vi "Read_Electrical_Variables.vi"(8 "error in (no error)":errorcluster, 11 "Modbus master in":refnum<class "Modbus Master.lvclass">) -> (0 "error out":errorcluster, 2 "Variables":sgl[](array[numeric]), 3 "Modbus master out":refnum<class "Modbus Master.lvclass">)   [LabVIEW 2019]
uses:
  <vilib>/Modbus/master/Modbus Master.lvclass
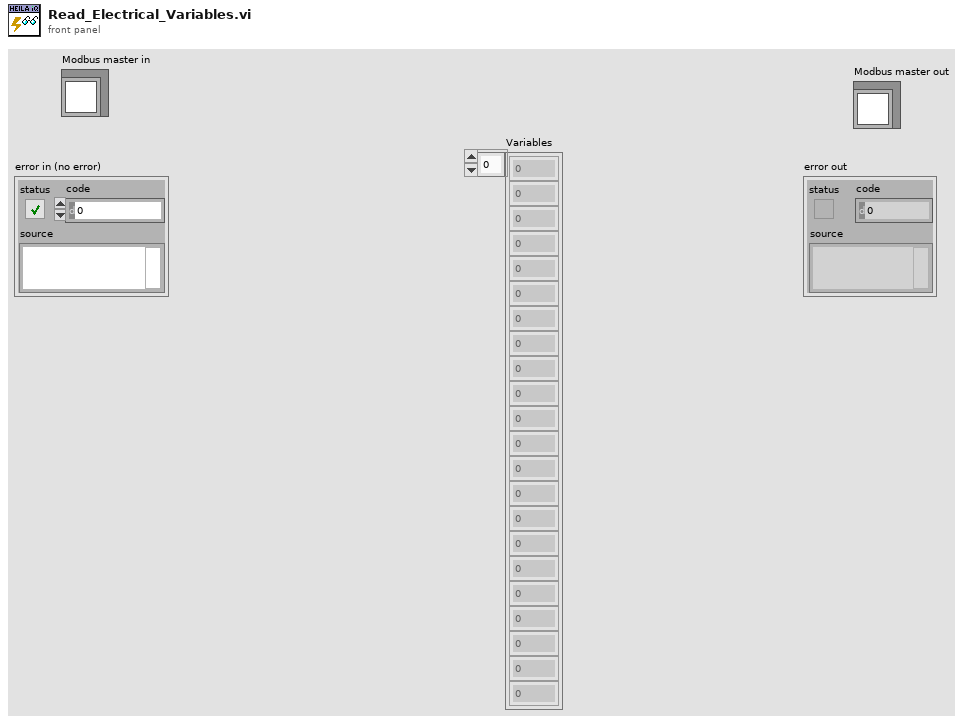
[diagram p1: front panel]
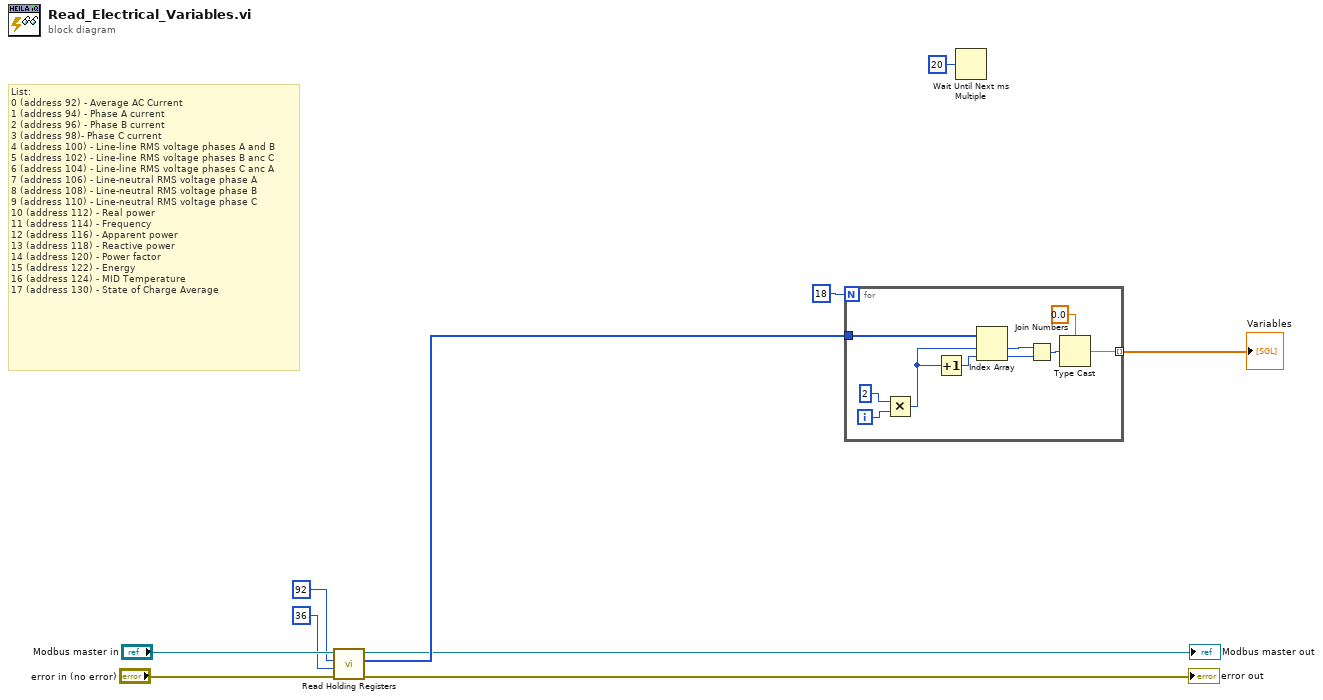
[diagram p0: block diagram]
diagram:
  # "List:\n0 (address 92) - Average AC Current\n1 (address 94) - Phase A current\n2 (address 96) - Phase B current\n3 (address 98)- Phase C current\n4 (address 100) - Line-line RMS voltage phases A and B\n5 (address 102) - Line-line RMS voltage phases B anc C\n6 (address 104) - Line-line RMS voltage phases C anc A\n7 (address 106) - Line-neutral RMS voltage phase A\n8 (address 108) - Line-neutral RMS voltage phase B\n9 (address 110) - Line-neutral RMS voltage phase C\n10 (address 112) - Real power\n11 (address 114) - Frequency\n12 (address 116) - Apparent power\n13 (address 118) - Reactive power\n14 (address 120) - Power factor\n15 (address 122) - Energy\n16 (address 124) - MID Temperature\n17 (address 130) - State of Charge Average"
  n1 = call-dynamic "Read Holding Registers.vi"("error in (no error)"="error in (no error)", "number of holding registers"=u16 36 ("starting address"), "starting address"=u16 92, "Modbus master in"="Modbus master in") -> ("error out"=→"error out":errorcluster, "register values"=w5:u16[], "Modbus master out"=→"Modbus master out":refnum<class "Modbus Master.lvclass">)  [unwired: 5 in]
  n2 = for {
    N: 18 -> [_]
    tunnel: [w16] -> w1 mode=indexing
    tunnel: w5 -> [w11]
    i -> [w15]
    n3 = Multiply(x=2, y=w15) -> (x*y=w12:i32)
    n4 = Increment(x=w12) -> (x+1=w13:i32)
    n5 = Index Array(array=w11, index #1=w12, index #2=w13) -> (element #1=w20:u16, element #2=w19:u16)
    n6 = Join Numbers(hi=w20, lo=w19) -> ((hi.lo)=w17:u32)
    n7 = Type Cast(type=sgl 0.0, x=w17) -> (*(type *) &x=w16:sgl)
  }
  "Variables" <- w1
  n8 = Wait Until Next ms Multiple(millisecond multiple=u32 20) -> ()  [unwired: 1 out]
